vi "Start Transaction.vi"(8 "error in":errorcluster, 11 "DB-ADO in":refnum<class "DB-ADO.lvclass">) -> (0 "error out":errorcluster, 3 "DB-ADO out":refnum<class "DB-ADO.lvclass">)   [LabVIEW 2014, in "hse-db.lvlib" / "DB-ADO.lvclass"]
doc: "Start a transaction to get sure all following SQL commands get executed or none."
uses:
  DB-ADO.lvclass
  DB-ADO.lvclass/DB-ADO.ctl
  DB-Engines/ADO-DB-Drivers/ADO-DB-Driver.lvlib
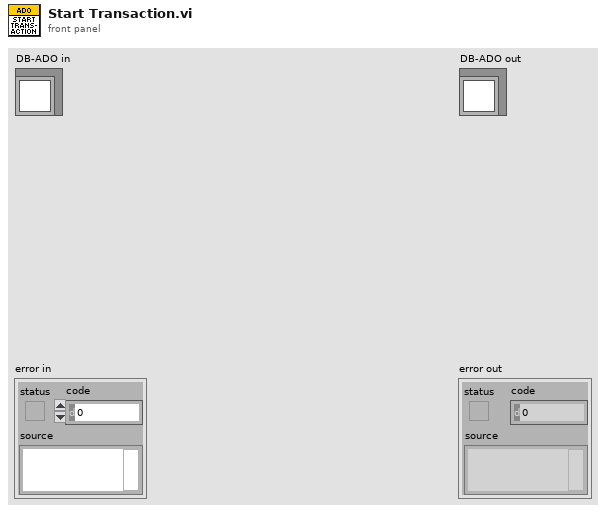
[diagram p1: front panel]
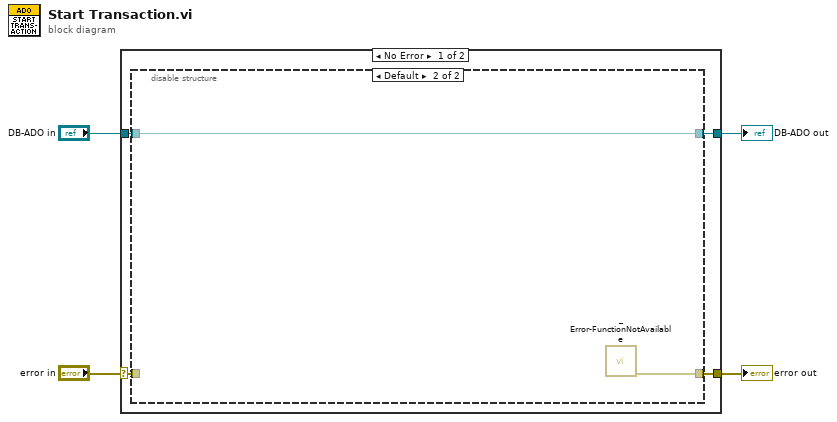
[diagram p0: block diagram]
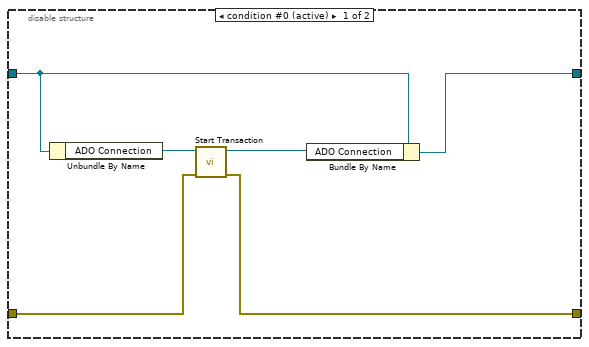
[diagram p2: hidden frame]
diagram:
  n1 = case shown="No Error" "error in" {
    selector: "error in" -> [w6 w18]
    tunnel: [w5 w18] -> w3
    tunnel: [w7 w17] -> w1
    tunnel: "DB-ADO in" -> [w8 w17]
    frame No Error {
      n2 = disable-structure shown="Default" {
        disable-tunnel: w8 -> [w12 w16]
        disable-tunnel: [w11 w16] -> w7
        disable-tunnel: w6 -> [w10 _]
        disable-tunnel: [w9 w15] -> w5
        frame condition #0 (active) {
          n3 = Unbundle By Name(w12) -> ("ADO Connection"=w14:refnum<k7>)
          n4 = call "Start Transaction.vi"("error in"=w10, "Connection In"=w14) -> ("error out"=w9:errorcluster, "Connection Out"=w13:refnum<k7>)  [unwired: 4 in]
          n5 = Bundle By Name(cluster=w12, "ADO Connection"=w13) -> (w11:refnum<class "DB-ADO.lvclass">)
        }
        frame condition #1 {
          n6 = call "_Error-FunctionNotAvailable.vi"() -> ("error out"=w15:errorcluster)  [unwired: 11 in]
        }
      }
    }
    frame Error {
    }
  }
  "error out" <- w3
  "DB-ADO out" <- w1
